vi "Terminal_Pressure_System_SaveToDB.vi"(8 "error in (no error)":errorcluster caption="错误输入（无错误）", 9 "时间标识":timestamp, 11 "设备信息":T1) -> (1 "error out":errorcluster)   [LabVIEW 2014]
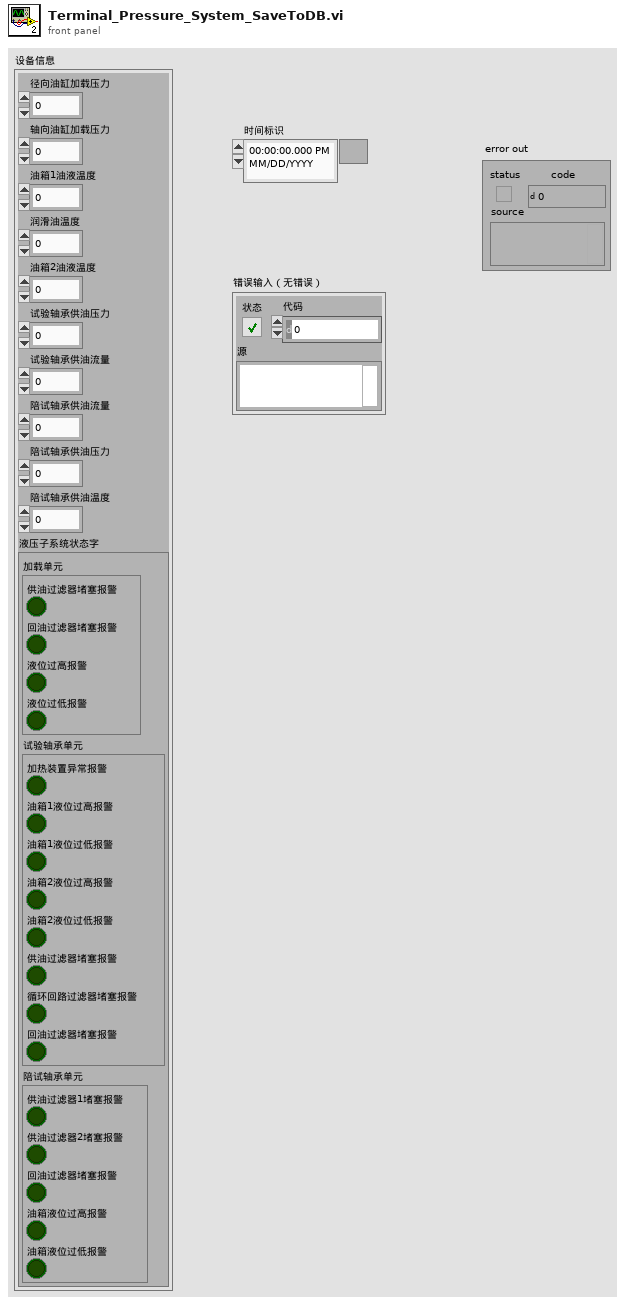
[diagram p1: front panel]
types:
  T1 = cluster{"径向油缸加载压力":u16, "轴向油缸加载压力":u16, "油箱1油液温度":u16, "润滑油温度":u16, "油箱2油液温度":u16, "试验轴承供油压力":u16, "试验轴承供油流量":u16, "陪试轴承供油流量":u16, "陪试轴承供油压力":u16, "陪试轴承供油温度":u16, "液压子系统状态字":cluster{"加载单元":cluster{"供油过滤器堵塞报警":bool, "回油过滤器堵塞报警":bool, "液位过高报警":bool, "液位过低报警":bool}, "试验轴承单元":cluster{"加热装置异常报警":bool, "油箱1液位过高报警":bool, "油箱1液位过低报警":bool, "油箱2液位过高报警":bool, "油箱2液位过低报警":bool, "供油过滤器堵塞报警":bool, "循环回路过滤器堵塞报警":bool, "回油过滤器堵塞报警":bool}, "陪试轴承单元":cluster{"供油过滤器1堵塞报警":bool, "供油过滤器2堵塞报警":bool, "回油过滤器堵塞报警":bool, "油箱液位过高报警":bool, "油箱液位过低报警":bool}}}
  T2 = cluster{"径向油缸加载压力":u16, "轴向油缸加载压力":u16, "油箱1油液温度":u16, "润滑油温度":u16, "油箱2油液温度":u16, "试验轴承供油压力":u16, "试验轴承供油流量":u16, "陪试轴承供油流量":u16, "陪试轴承供油压力":u16, "陪试轴承供油温度":u16}
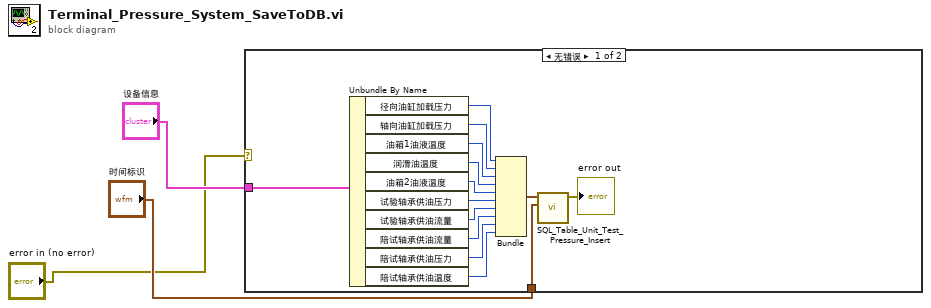
[diagram p0: block diagram]
diagram:
  n1 = case shown="无错误" "error in (no error)" {
    tunnel: "时间标识" -> [w6 _]
    tunnel: "设备信息" -> [w5 _]
    frame No Error {
      n2 = Unbundle By Name(w5) -> ("径向油缸加载压力"=w17:u16, "轴向油缸加载压力"=w16:u16, "油箱1油液温度"=w15:u16, "润滑油温度"=w14:u16, "油箱2油液温度"=w13:u16, "试验轴承供油压力"=w12:u16, "试验轴承供油流量"=w11:u16, "陪试轴承供油流量"=w10:u16, "陪试轴承供油压力"=w9:u16, "陪试轴承供油温度"=w8:u16)
      n3 = Bundle("径向油缸加载压力"=w17, "轴向油缸加载压力"=w16, "油箱1油液温度"=w15, "润滑油温度"=w14, "油箱2油液温度"=w13, "试验轴承供油压力"=w12, "试验轴承供油流量"=w11, "陪试轴承供油流量"=w10, "陪试轴承供油压力"=w9, "陪试轴承供油温度"=w8) -> (w7:T2)  [unwired: 1 in]
      n4 = call "SQL_Table_Unit_Test_Pressure_Insert.vi"("时间标识"=w6, "液压子系统数据"=w7) -> ("error out"=→"error out":errorcluster)  [unwired: 9 in]
    }
    frame Error {
    }
  }
